vi "Test PyBaMM Wrapper.vi"() -> ()   [LabVIEW 2023, in "Battery.lvclass"]
uses:
  Battery.lvclass
  Simulation Parameters.ctl
panel:
  out "state_of_charges":dbl[](array[numeric])
  in  "Simulation Parameters":T1={"# RC Pairs"=1, "R0 (Ohm)"=0.0015, "R1 (Ohm)"=0.001, "C1 (Farad)"=2500.0, "R2 (Ohm)"=0.0008, "C2 (Farad)"=40000.0, "Nominal Capacity (Ah)"=5.0, "Upper Cutoff Voltage"=4.2, "Lower Cutoff Voltage"=3.0, "Coulombic Efficiency"=3.0} {"# RC Pairs" min=1 max=2}
  out "terminal_voltages":dbl[](array[numeric])
  in  "time_step_s":dbl=600.0 format="%#_13g"
  in  "current_A":dbl=5.0 format="%#_13g"
  in  "number of simulation steps":i32=100
  out "simulation loaded":bool
  out "XY Graph":cluster{dbl[], dbl[]}[](graph)
  in  "module path":path=path "C:/Repo/hps17k-panel/src/Python/hps17k-pybamm-wrapper.py"
  out "error out":errorcluster
  in  "venv path":path=path "C:/Repo/volta-control-suite/venv"
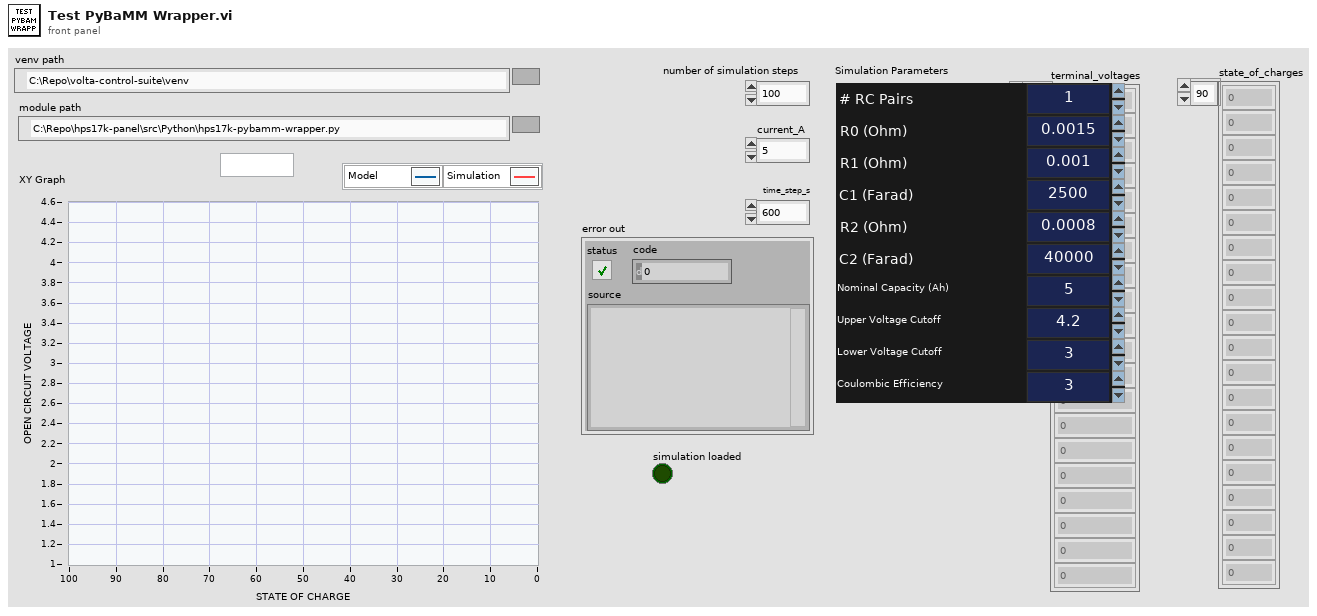
[diagram p1: front panel]
types:
  T1 = typedef "Battery.lvclass/Simulation Parameters.ctl" = cluster{"# RC Pairs":u8, "R0 (Ohm)":dbl, "R1 (Ohm)":dbl, "C1 (Farad)":dbl, "R2 (Ohm)":dbl, "C2 (Farad)":dbl, "Nominal Capacity (Ah)":dbl, "Upper Cutoff Voltage":dbl, "Lower Cutoff Voltage":dbl, "Coulombic Efficiency":dbl}
  T2 = cluster{"SOC OCV Curve":dbl[], "SOC OCV Curve":dbl[]}
  T3 = cluster{"SOC OCV Curve":dbl[], "SOC OCV Curve":dbl[]}[]
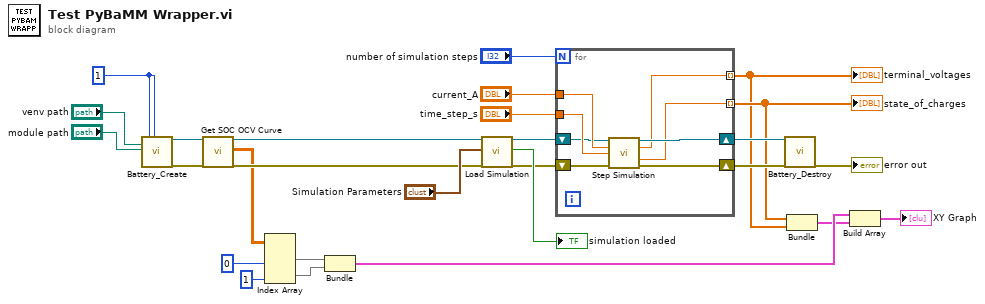
[diagram p0: block diagram]
diagram:
  w1 = u16 1 ("# Cells in Series")
  n1 = call "Battery_Create.vi"("Python venv"="venv path", "Python module"="module path", "# Cells in Series"=w1, "# Cells in Parallel"=w1) -> ("reference out"=w3:refnum<class "Battery.lvclass">, "Error Out"=w2:errorcluster)  [unwired: 13 in, 1 out]
  n2 = call-dynamic "Get SOC OCV Curve.vi"("reference in"=w3, "Error In"=w2) -> ("reference out"=w14:refnum<class "Battery.lvclass">, "SOC OCV Curve"=w12:dbl[][], "Error Out"=w15:errorcluster)  [unwired: 15 in]
  n3 = Index Array(array=w12, index (col) #1=0 ("disabled index (col)"), index (col) #2=1 ("disabled index (col)")) -> (element #1=w9:dbl[], element #2=w8:dbl[])  [unwired: 2 in]
  n4 = Bundle("SOC OCV Curve"=w9, "SOC OCV Curve"=w8) -> (w7:T2)  [unwired: 1 in]
  n5 = call-dynamic "Load Simulation.vi"("reference in"=w14, "Simulation Parameters"="Simulation Parameters", "Error In"=w15) -> ("reference out"=w18:refnum<class "Battery.lvclass">, "simulation loaded"=→"simulation loaded":bool, "Error Out"=w19:errorcluster)  [unwired: 14 in]
  n6 = for {
    N: "number of simulation steps" -> [_]
    shift-right: [w32] -> w17
    shift-left: w19 -> [w35]
    tunnel: "current_A" -> [w34]
    tunnel: "time_step_s" -> [w33]
    tunnel: [w28] -> w4 mode=indexing
    shift-right: [w30] -> w16
    shift-left: w18 -> [w31]
    tunnel: [w29] -> w5 mode=indexing
    n7 = call-dynamic "Step Simulation.vi"("reference in"=w31, "current_A"=w34, "time_step_S"=w33, "Error In"=w35) -> ("reference out"=w30:refnum<class "Battery.lvclass">, "terminal voltage"=w28:dbl, "state of charge"=w29:dbl, "Error Out"=w32:errorcluster)  [unwired: 7 in, 1 out]
  }
  "terminal_voltages" <- w4
  "state_of_charges" <- w5
  n8 = call-dynamic "Battery_Destroy.vi"("reference in"=w16, "Error In"=w17) -> ("Error Out"=→"error out":errorcluster)  [unwired: 16 in, 1 out]
  n9 = Bundle(w5, w4) -> (w6:cluster{dbl[], dbl[]})  [unwired: 1 in]
  n10 = Build Array(w7, w6) -> (→"XY Graph":T3)
